vi "Decide next action Rate base_test.vi"(7 "Seek Function":enum16{"Rate based", "Ploarization(avg) based"}(ring), 8 "error in (no error)":errorcluster, 9 "Seek?":bool, 10 "Seek positive polarization?":bool, 11 "Automation in":refnum<class "Automation.lvclass">) -> (0 "error out":errorcluster, 1 "Should reseek?":bool, 2 "Decision":T1, 3 "Automation out":refnum<class "Automation.lvclass">, 4 "average Polarization":dbl format="%0.2f", 6 "mean rate":dbl format="%.9f")   [LabVIEW 2019, in "Automation.lvclass"]
uses:
  Automation.lvclass
  Automatic mode/Controller decision.ctl
  Automation.lvclass/Automation.ctl
  <vilib>/Analysis/baseanly.llb/Mean (DBL).vi
  <vilib>/gmath/NI_Gmath.lvlib
  <vilib>/Analysis/NI_AALBase.lvlib
panel:
  in  "\"Steady\" polarization spread":dbl=0.002
  out "Last rate":dbl
  out "Slopes":dbl[](array[numeric])
  out "Polarizations":dbl[](array[numeric])
  out "spread value":dbl
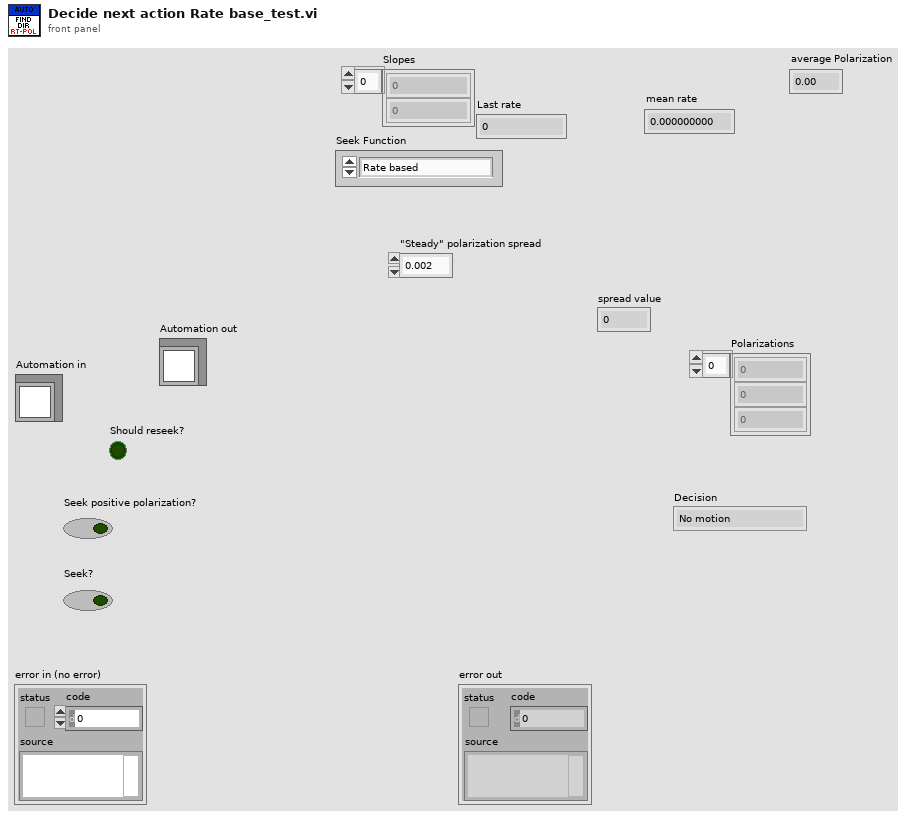
[diagram p1: front panel]
types:
  T1 = typedef "Controller decision.ctl" = enum16{"No motion", "Switch direction", "Keep current direction"}
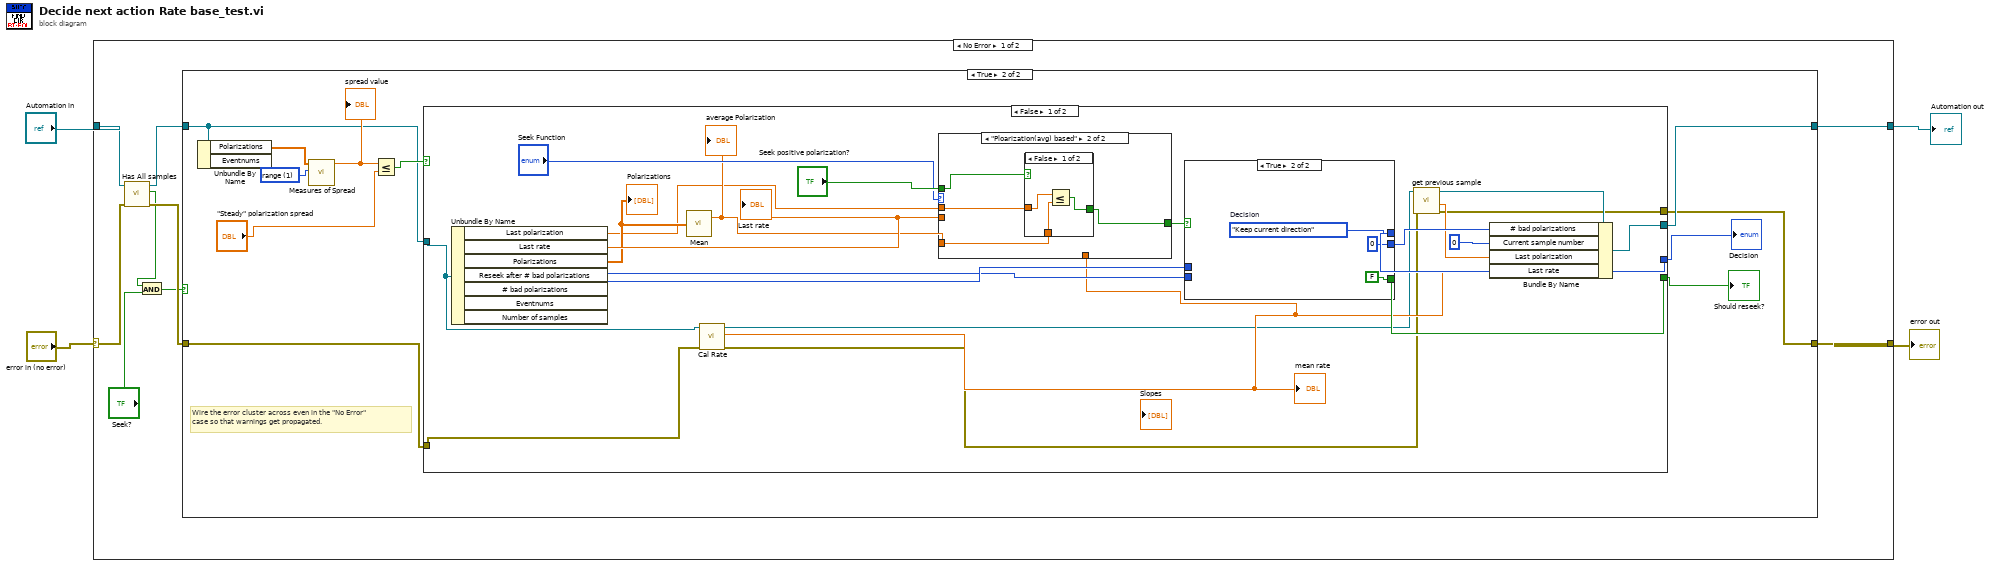
[diagram p0: block diagram]
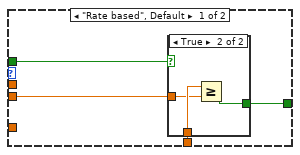
[diagram p3: hidden frame]
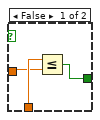
[diagram p4: hidden frame]
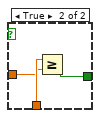
[diagram p5: hidden frame]
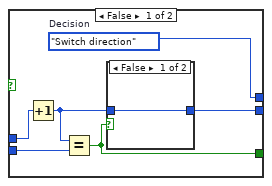
[diagram p6: hidden frame]
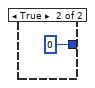
[diagram p7: hidden frame]
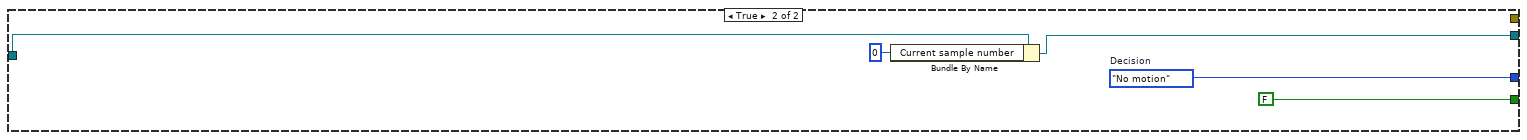
[diagram p8: hidden frame]
diagram:
  n1 = case shown="No Error" "error in (no error)" {
    selector: "error in (no error)" -> [w10 w86]
    tunnel: [w12 w86] -> w3
    tunnel: [w13 w85] -> w1
    tunnel: "Automation in" -> [w11 w85]
    frame No Error {
      n2 = call "Has All samples.vi"("error in (no error)"=w10, "Automation in"=w11) -> ("error out"=w9:errorcluster, "Has all samples?"=w6:bool, "Automation out"=w8:refnum<class "Automation.lvclass">)  [unwired: 7 in]
      n3 = And(x=w6, y="Seek?") -> (x .and. y?=w7:bool)
      n4 = case shown="True" w7 {
        tunnel: w8 -> [w14 w23]
        tunnel: [w14 w21] -> w13
        tunnel: [w15 w18] -> w12
        tunnel: w9 -> [w15 w17]
        frame False {
        }
        frame True {
          w26 = 1 items=["standard deviation", "range", "mean absolute deviation", "interquartile range"] ("type")
          # "Wire the error cluster across even in the \"No Error\"\ncase so that warnings get propagated."
          n5 = Unbundle By Name(w23) -> ("Polarizations"=w22:dbl[])  [unwired: 1 out]
          n6 = call <vilib>:"Measures of Spread.vi"("type"=w26, "x array"=w22) -> ("spread value"=w25:dbl)  [unwired: 8 in, 1 out]
          "spread value" <- w25
          n7 = Less Or Equal?(x=w25, y="\"Steady\" polarization spread") -> (x <= y?=w24:bool)
          n8 = case shown="False" w24 {
            tunnel: [w44 w81] -> w21
            tunnel: [w48 w83] -> w20
            tunnel: [w45 FALSE] -> w19
            tunnel: w23 -> [w32 w82]
            tunnel: [w39 _] -> w18
            tunnel: w17 -> [w35 _]
            frame False {
              n9 = Unbundle By Name(w32) -> ("Last polarization"=w27:dbl, "Last rate"=w37:dbl, "Polarizations"=w29:dbl[], "Reseek after # bad polarizations"=w43:u32, "# bad polarizations"=w46:u32)  [unwired: 2 out]
              "Polarizations" <- w29
              "Last rate" <- w37
              n10 = call-poly <vilib>:"Mean.vi"("X"=w29) -> ("mean"=w28:dbl)  [unwired: 1 out]
              "average Polarization" <- w28
              n11 = call "Cal Rate.vi"("error in (no error)"=w35, "Automation in"=w32) -> ("error out"=w34:errorcluster, "mean Rate"=w36:dbl, "Automation out"=w33:refnum<class "Automation.lvclass">)  [unwired: 7 in]
              "mean rate" <- w36
              n12 = case shown="\"Ploarization(avg) based\"" "Seek Function" {
                tunnel: [w52 w62] -> w38
                tunnel: w37 -> [w51 _]
                tunnel: w36 -> [w50 _]
                tunnel: "Seek positive polarization?" -> [w49 w61]
                tunnel: w28 -> [_ w60]
                tunnel: w27 -> [_ w59]
                frame "Rate based", Default {
                  n13 = case shown="True" w49 {
                    tunnel: [w55 w58] -> w52
                    tunnel: w50 -> [w54 w57]
                    tunnel: w51 -> [w53 w56]
                    frame False {
                      n14 = Less Or Equal?(x=w54, y=w53) -> (x <= y?=w55:bool)
                    }
                    frame True {
                      n15 = Greater Or Equal?(x=w57, y=w56) -> (x >= y?=w58:bool)
                    }
                  }
                }
                frame "Ploarization(avg) based" {
                  n16 = case shown="False" w61 {
                    tunnel: [w65 w68] -> w62
                    tunnel: w60 -> [w63 w67]
                    tunnel: w59 -> [w64 w66]
                    frame False {
                      n17 = Less Or Equal?(x=w64, y=w63) -> (x <= y?=w65:bool)
                    }
                    frame True {
                      n18 = Greater Or Equal?(x=w67, y=w66) -> (x >= y?=w68:bool)
                    }
                  }
                }
              }
              n19 = case shown="True" w38 {
                tunnel: [w69 w77] -> w48
                tunnel: [w71 u32 0] -> w47
                tunnel: w46 -> [w74 _]
                tunnel: [w72 FALSE] -> w45
                tunnel: w43 -> [w73 _]
                frame False {
                  w69 = Controller_decision."Switch direction"  # Decision
                  n20 = Increment(x=w74) -> (x+1=w70:u32)
                  n21 = Equal?(x=w70, y=w73) -> (x = y?=w72:bool)
                  n22 = case shown="False" w72 {
                    tunnel: [w75 0] -> w71
                    tunnel: w70 -> [w75 _]
                    frame False {
                    }
                    frame True {
                    }
                  }
                }
                frame True {
                  w77 = Controller_decision."Keep current direction"  # Decision
                }
              }
              n23 = call "get previous sample.vi"("error in (no error)"=w34, "Automation in"=w33) -> ("error out"=w39:errorcluster, "Polarization"=w40:dbl, "Automation out"=w41:refnum<class "Automation.lvclass">)  [unwired: 6 in, 1 out]
              n24 = Bundle By Name(cluster=w41, "# bad polarizations"=w47, "Current sample number"=0, "Last polarization"=w40, "Last rate"=w36) -> (w44:refnum<class "Automation.lvclass">)
            }
            frame True {
              w83 = Controller_decision."No motion"  # Decision
              n25 = Bundle By Name(cluster=w82, "Current sample number"=0) -> (w81:refnum<class "Automation.lvclass">)
            }
          }
          "Decision" <- w20
          "Should reseek?" <- w19
        }
      }
    }
    frame Error {
    }
  }
  "error out" <- w3
  "Automation out" <- w1
